vi "exp4_cw.vi"() -> ()   [LabVIEW 2022 SP3]
uses:
  <vilib>/Analysis/3filter.llb/Filter Passband Type.ctl
  <vilib>/Analysis/2dsp.llb/Real FFT.vi
  <vilib>/Analysis/3filter.llb/Butterworth Filter (DBL).vi
  <vilib>/Analysis/NI_AALBase.lvlib
  <vilib>/Analysis/NI_AALPro.lvlib
panel:
  out "滤波后信号频谱":dbl[](graph)
  out "滤波后信号":dbl[](graph)
  out "输入信号频谱":dbl[](graph)
  out "输入信号":dbl[](graph)
  in  "采样数":i32
  in  "信号频率":dbl
  in  "采样频率 (fs)":dbl
  in  "截止频率":dbl(slide) scale=0.0..200.0
  in  "阶数":i32(slide) min=0 max=5 step=1 scale=0.0..5.0
  in  "停止":bool
  in  "滤波器":enum16{"Butterworth", "Chebyshev"}(ring)
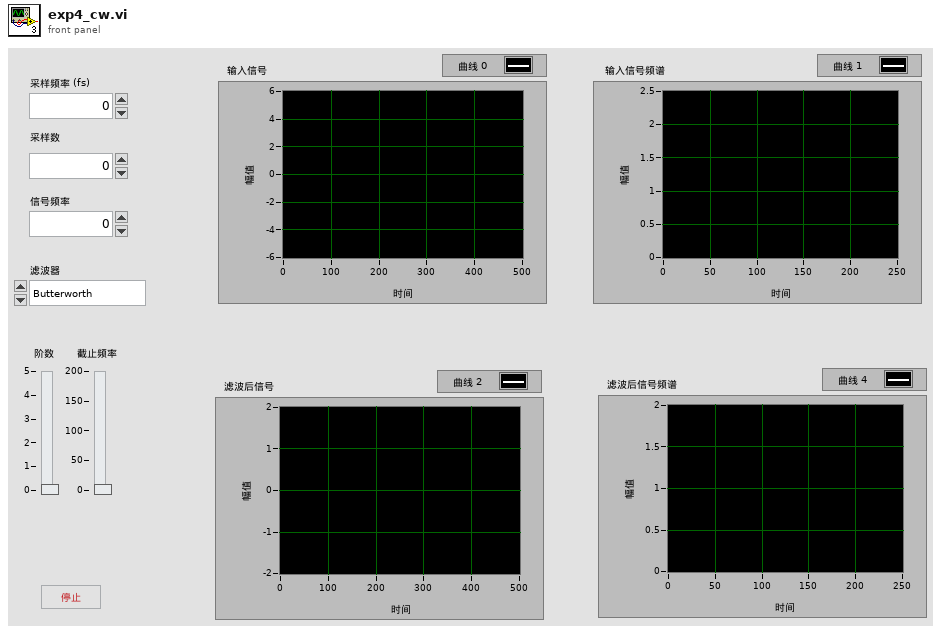
[diagram p1: front panel]
types:
  T1 = typedef "NI_AALBase.lvlib/Filter Passband Type.ctl" = enum32{"Lowpass", "Highpass", "Bandpass", "Bandstop"}
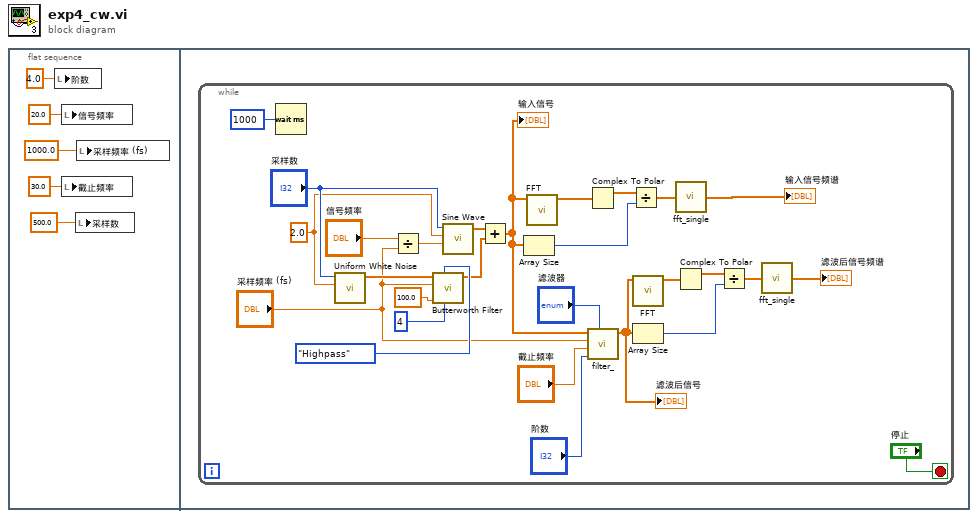
[diagram p0: block diagram]
diagram:
  n1 = flat-sequence {
    frame #0 {
      n2 = local write "阶数"(4.0) -> ()
      n3 = local write "信号频率"(20.0) -> ()
      n4 = local write "截止频率"(30.0) -> ()
      n5 = local write "采样数"(500.0) -> ()
      n6 = local write "采样频率 (fs)"(1000.0) -> ()
    }
    frame #1 {
      n7 = while {
        stop <- "停止" stop-if-true
        w15 = 2.0 ("幅值 (V)")
        n8 = Wait (ms)(milliseconds to wait=u32 1000 ("等待时间（毫秒）")) -> ()  [unwired: 1 out]
        n9 = call <vilib>:"Uniform White Noise.vi"("amplitude"=w15, "samples"="采样数") -> ("uniform white noise"=w23:dbl[])  [unwired: 8 in, 1 out]
        n10 = Divide(x="信号频率", y="采样频率 (fs)") -> (x/y=w31:dbl)
        n11 = call-poly <vilib>:"Butterworth Filter.vi"("order"=4, "filter type"=Filter_Passband_Type."Highpass", "low cutoff freq: fl"=100.0, "sampling freq: fs"="采样频率 (fs)", "X"=w23) -> ("Filtered X"=w20:dbl[])  [unwired: 3 in, 1 out]
        n12 = call <vilib>:"Sine Wave.vi"("samples"="采样数", "amplitude"=w15, "frequency"=w31) -> ("sine wave"=w21:dbl[])  [unwired: 2 in, 2 out]
        n13 = Add(x=w21, y=w20) -> (x+y=w9:dbl[])
        "输入信号" <- w9
        n14 = Array Size(array=w9) -> (size(s)=w28:i32)
        n15 = call-poly <vilib>:"FFT.vi"("X"=w9) -> ("FFT {X}"=w30:cdb[])  [unwired: 9 in, 1 out]
        n16 = Complex To Polar(r * e^(i*theta)=w30) -> (r=w29:dbl[])  [unwired: 1 out]
        n17 = call "filter_.vi"("滤波方法"="滤波器", "阶数"="阶数", "截止频率"="截止频率", "采样频率 (fs)"="采样频率 (fs)", "输入信号"=w9) -> ("输出信号"=w7:dbl[])  [unwired: 6 in]
        "滤波后信号" <- w7
        n18 = Divide(x=w29, y=w28) -> (x/y=w16:dbl[])
        n19 = call-poly <vilib>:"FFT.vi"("X"=w7) -> ("FFT {X}"=w27:cdb[])  [unwired: 9 in, 1 out]
        n20 = Array Size(array=w7) -> (size(s)=w25:i32)
        n21 = call "fft_single.vi"("双边fft"=w16) -> ("单边fft"=→"输入信号频谱":dbl[])
        n22 = Complex To Polar(r * e^(i*theta)=w27) -> (r=w26:dbl[])  [unwired: 1 out]
        n23 = Divide(x=w26, y=w25) -> (x/y=w10:dbl[])
        n24 = call "fft_single.vi"("双边fft"=w10) -> ("单边fft"=→"滤波后信号频谱":dbl[])
      }
    }
  }
